vi "CreatePrivateEvents.vi"(8 "error in (no error)":errorcluster, 11 "MeasurementSMO":refnum<class "MeasurementSMO.lvclass">) -> (0 "error out":errorcluster, 3 "MeasurementSMO out":refnum<class "MeasurementSMO.lvclass">)   [LabVIEW 2019, in "MeasurementSMO.lvclass"]
doc: "---------------------------------------------------------------\nJKI State Machine Objects™\nhttp://jki.net/state-machine-objects/\nCopyright (C) 2005-2015, JKI <info@jki.net>\nALL RIGHTS RESERVEDJKI State Machine Objects (SMO) 1.0.0.4\nJKI - JKI\nCopyright (c) 2015, JKI"
uses:
  MeasurementSMO.lvclass
  Typedefs/PrivateEvents--MeasurementSMO.IV Run--Local.ctl
  Typedefs/PrivateEvents--MeasurementSMO.IV Status--Local.ctl
  MeasurementSMO.lvclass/MeasurementSMO.ctl
  <vilib>/JKI/JKI SMO/SMO/SMO.lvclass
panel:
  # "For instructions on how to use the JKI State Machine Objects, examples and video tutorials, visit:\nhttp://jki.net/state-machine-objects/\n\nJKI State Machine Objects™\nhttp://jki.net/state-machine-objects/\nCopyright (C) 2005-2015, JKI <info@jki.net>\nALL RIGHTS RESERVED"
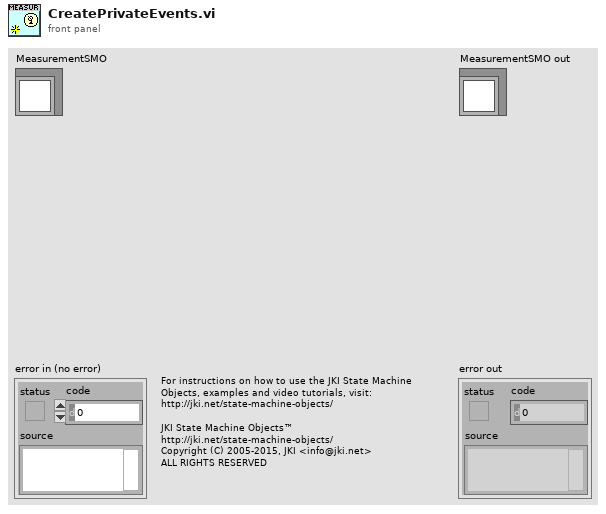
[diagram p1: front panel]
types:
  T1 = typedef "MeasurementSMO.lvclass/PrivateEvents--MeasurementSMO.IV Status--Local.ctl" = cluster{"Return":refnum<notifier>}
  T2 = typedef "MeasurementSMO.lvclass/PrivateEvents--MeasurementSMO.IV Run--Local.ctl" = cluster{"Pattern":enum16{"Ramp /", "Ramp /\\", "Smooth Ramp _/", "Smooth Ramp _/\\_", "Frequency"}, "Cycles":dbl, "Rate":dbl, "End":dbl, "Start":dbl}
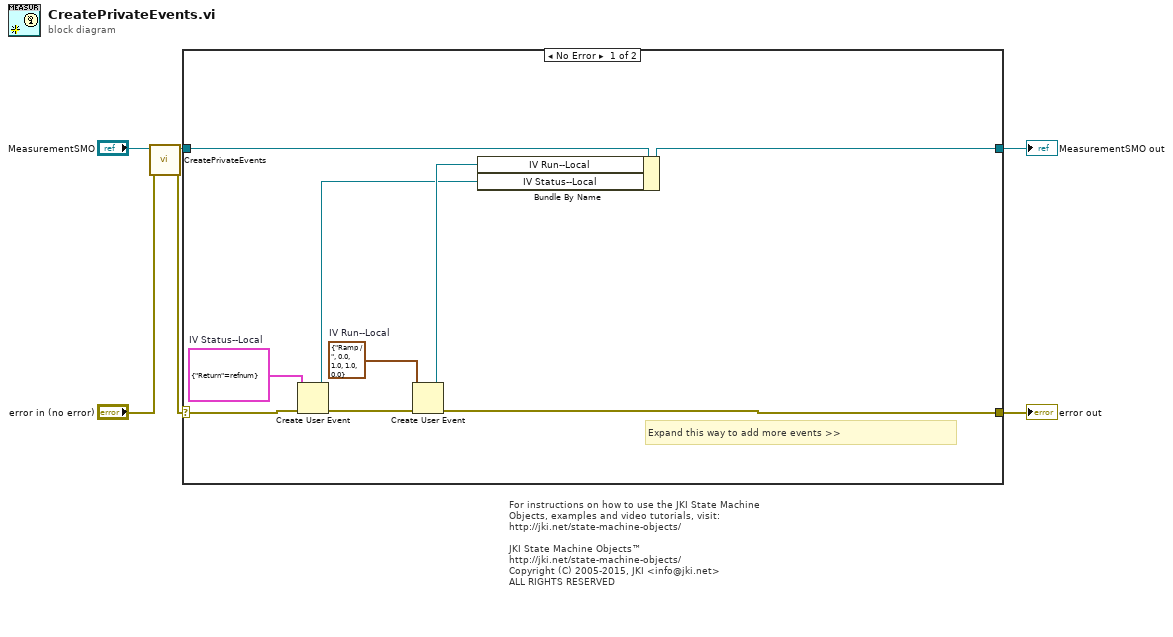
[diagram p0: block diagram]
diagram:
  # "For instructions on how to use the JKI State Machine Objects, examples and video tutorials, visit:\nhttp://jki.net/state-machine-objects/\n\nJKI State Machine Objects™\nhttp://jki.net/state-machine-objects/\nCopyright (C) 2005-2015, JKI <info@jki.net>\nALL RIGHTS RESERVED"
  n1 = call-parent "CreatePrivateEvents.vi"("error in (no error)"="error in (no error)", "SMO"="MeasurementSMO") -> ("error out"=w1:errorcluster, "SMO out"=w3:refnum<class "MeasurementSMO.lvclass">)  [unwired: 8 in]
  n2 = case shown="No Error" w1 {
    selector: w1 -> [w14 w17]
    tunnel: [w12 w17] -> w5
    tunnel: [w13 w16] -> w6
    tunnel: w3 -> [w15 w16]
    frame No Error {
      w8 = T1 {"Return"=refnum}  # IV Status--Local
      w11 = T2 {"Pattern"=enum."Ramp /", "Cycles"=0.0, "Rate"=1.0, "End"=1.0, "Start"=0.0}  # IV Run--Local
      # "Expand this way to add more events >>"
      n3 = Create User Event(user event datatype=w8, error in=w14) -> (user event=w7:refnum<user-event>, error out=w9:errorcluster)
      n4 = Create User Event(user event datatype=w11, error in=w9) -> (user event=w10:refnum<user-event>, error out=w12:errorcluster)
      n5 = Bundle By Name(cluster=w15, "IV Run--Local"=w10, "IV Status--Local"=w7) -> (w13:refnum<class "MeasurementSMO.lvclass">)
    }
    frame Error {
    }
  }
  "error out" <- w5
  "MeasurementSMO out" <- w6
